vi "Stop ZeroMQ VIs.vi"(8 "error in (no error)":errorcluster, 11 "Header content in":refnum<class "Header content.lvclass">) -> (0 "error out":errorcluster, 3 "Header content out":refnum<class "Header content.lvclass">)   [LabVIEW 2018, in "Header content.lvclass"]
uses:
  Header content.lvclass
  Header content.lvclass/Header content.ctl
  Server/Server.lvclass
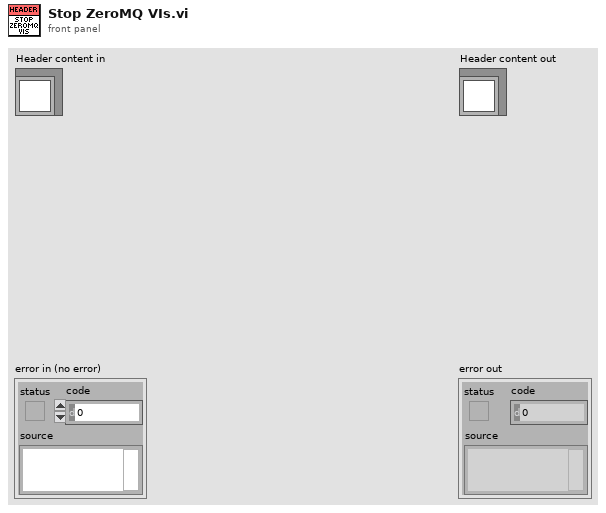
[diagram p1: front panel]
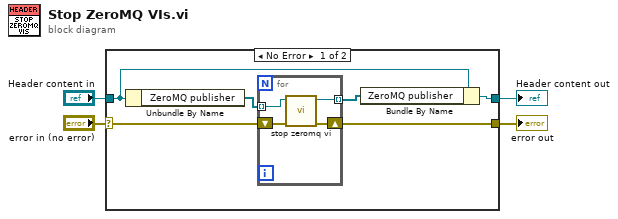
[diagram p0: block diagram]
diagram:
  n1 = case shown="No Error" "error in (no error)" {
    selector: "error in (no error)" -> [w5 w16]
    tunnel: [w9 w16] -> w3
    tunnel: [w7 w15] -> w1
    tunnel: "Header content in" -> [w8 w15]
    frame No Error {
      n2 = Unbundle By Name(w8) -> ("ZeroMQ publisher"=w10:refnum<class "Server.lvclass">[])
      n3 = for {
        tunnel: w10 -> [w14] mode=indexing
        shift-right: [w13] -> w9
        shift-left: w5 -> [w11]
        tunnel: [w12] -> w6 mode=indexing
        n4 = call "stop zeromq vi.vi"("error in (no error)"=w11, "Server in"=w14) -> ("error out"=w13:errorcluster, "Server out"=w12:refnum<class "Server.lvclass">)  [unwired: 8 in]
      }
      n5 = Bundle By Name(cluster=w8, "ZeroMQ publisher"=w6) -> (w7:refnum<class "Header content.lvclass">)
    }
    frame Error {
    }
  }
  "error out" <- w3
  "Header content out" <- w1
